vi "4461 - Create IO Channels Parallel Uneven array.vi"(0 "sample mode":i32(ring)=10178 items=["Finite Samples"=10178, "Continuous Samples"=10123], 1 "Channels: Lockin":T1={"REF f (Hz)"=[0.4, 0.4], "REF phi (deg)"=[0.0, 0.0]} {"REF phi (deg)" format="%#_3g"}, 6 "error in":errorcluster, 7 "AI Buffer Size (S)":i32=10, 8 "sampling info":cluster{"Fs":dbl, "#s":dbl}, 9 "AO":T2={"AO amp (V)"=[0.1, 0.09, 0.08, 0.07, 0.06, 0.05, 0.04, 0.03], "AO DC (V)"=[0.0, 0.0, 0.0, 0.0, 0.0, 0.0, 0.0, 0.0], "AO f (Hz)"=[13.0, 13.0, 13.0, 13.0, 13.0, 13.0, 13.0, 13.0], "AO phi (deg)"=[0.0, 0.0, 0.0, 0.0, 0.0, 0.0, 0.0, 0.0], "function"=[enum."Sine Wave", enum."Sine Wave", enum."Sine Wave", enum."Sine Wave", enum."Sine Wave", enum."Sine Wave", enum."Sine Wave", enum."Sine Wave"]} {"AO DC (V)" format="%#_6p"; "AO amp (V)" format="%#_6p"}, 10 "AO Configuration":T3(array[cluster]), 11 "AI Configuration":T4(array[cluster])) -> (2 "AO Task":refnum<k21>[](array[refnum]), 3 "AI task":refnum<k21>[](array[refnum]), 4 "error out":errorcluster, 5 "phase log":dbl[](array[numeric])=[0.99999999999938, 0.99999999999938])   [LabVIEW 2016]
uses:
  <vilib>/DAQmx/write.llb/DAQmx Write (Analog 1D Wfm NChan NSamp).vi
  <vilib>/DAQmx/read.llb/DAQmx Read (Analog 1D Wfm NChan NSamp).vi
  <vilib>/DAQmx/create/channels.llb/DAQmx Create Channel (AI-Voltage-Basic).vi
  <vilib>/DAQmx/configure/timing.llb/DAQmx Timing (Sample Clock).vi
  <vilib>/DAQmx/create/channels.llb/DAQmx Create Channel (AO-Voltage-Basic).vi
  <vilib>/DAQmx/miscellaneous.llb/DAQmx Fill In Error Info.vi
  <resource>/objmgr/daqmx.rc
panel:
  out "RefClk.Src":tag
  out "#samp":dbl
  in  "AI.FilterDelay":dbl
  in  "AI.Gain":dbl
  in  "input terminal configuration":i32(ring)=-1 items=["default"=-1, "RSE"=10083, "NRSE"=10078, "Differential"=10106, "Pseudodifferential"=12529]
  in  "output terminal configuration":i32(ring)=-1 items=["Default"=-1, "RSE"=10083, "Differential"=10106, "Pseudodifferential"=12529]
  out "SampClk.Timebase.Rate":dbl
  out "SampQuant.SampPerChan":dbl
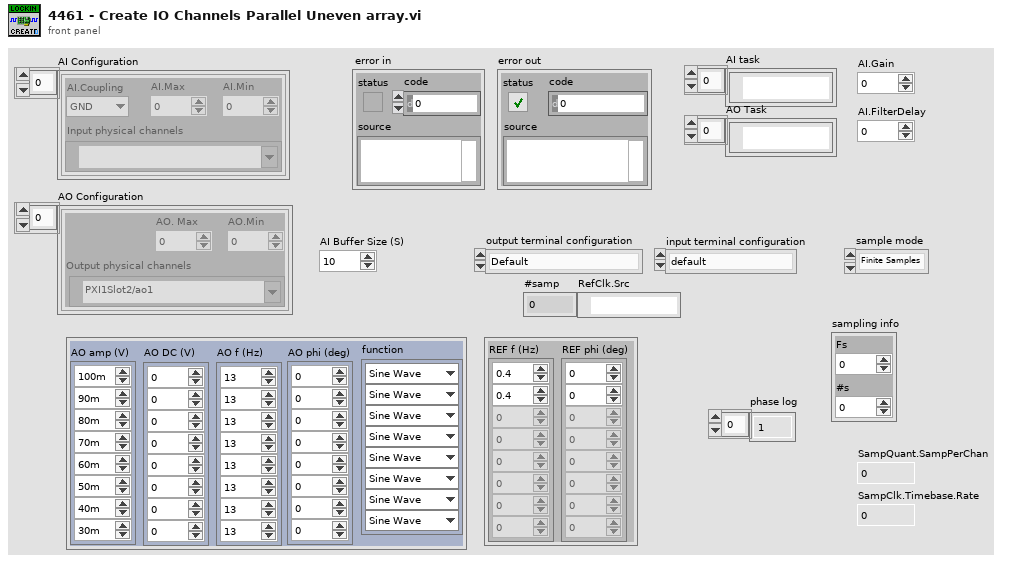
[diagram p1: front panel]
types:
  T1 = cluster{"REF f (Hz)":dbl[], "REF phi (deg)":dbl[]}
  T2 = cluster{"AO amp (V)":dbl[], "AO DC (V)":dbl[], "AO f (Hz)":dbl[], "AO phi (deg)":dbl[], "function":enum16{"Sine Wave", "Triangle Wave", "Square Wave", "Sawtooth Wave"}[]}
  T3 = cluster{"Output physical channels":tag, "AO. Max":dbl, "AO.Min":dbl}[]
  T4 = cluster{"AI.Coupling":enum16{"AC", "DC", "GND"}, "AI.Max":dbl, "AI.Min":dbl, "Input physical channels":tag}[]
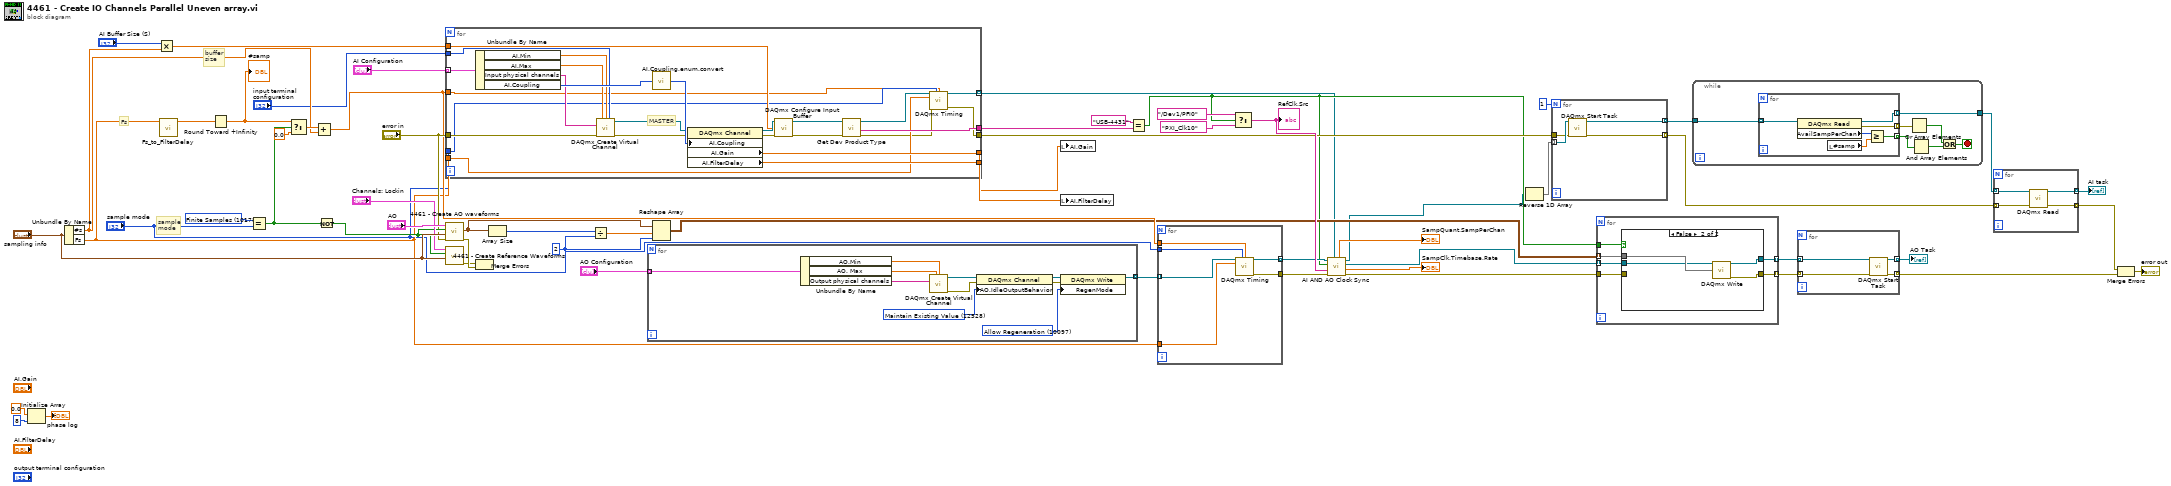
[diagram p0: block diagram]
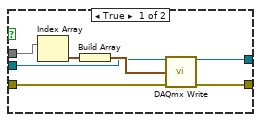
[diagram p2: hidden frame]
diagram:
  w14 = 2 ("y")
  w53 = 10178 items=["Finite Samples"=10178, "Continuous Samples"=10123] ("sample mode 2")
  # "Fs"
  # "sample\nmode"
  # "buffer\nsize"
  n1 = Initialize Array(0.0 ("element"), 8 ("dimension size")) -> (→"phase log":dbl[])
  n2 = Unbundle By Name("sampling info") -> ("#s"=w50:dbl, "Fs"=w29:dbl)
  n3 = Multiply(x="AI Buffer Size (S)", y=w50) -> (x*y=w36:dbl)
  n4 = call "Fs_to_FilterDelay.vi"("Fs"=w29) -> ("Total Filter Delay (samples)"=w56:dbl)  [unwired: 10 in]
  n5 = Round Toward +Infinity(x=w56) -> (ceil(x): smallest int >= x=w46:dbl)
  "#samp" <- w46
  n6 = Equal?(x=w53, y="sample mode") -> (x = y?=w48:bool)
  n7 = Select(t=w46, s=w48, f=0.0) -> (s? t:f=w54:dbl)
  n8 = Add(x=w54, y=w50) -> (x+y=w30:dbl)
  n9 = Not(x=w48) -> (.not. x?=w47:bool)
  n10 = for {
    tunnel: "AI Configuration" -> [w78] mode=indexing
    tunnel: "input terminal configuration" -> [w77]
    tunnel: [w76] -> w39
    tunnel: [w75] -> w38
    tunnel: "error in" -> [w74]
    tunnel: [w61] -> w7
    tunnel: w36 -> [w72]
    tunnel: [w68] -> w35
    tunnel: w29 -> [w66]
    tunnel: "sample mode" -> [w65]
    tunnel: w30 -> [w64]
    tunnel: [w63] -> w5 mode=indexing
    # "MASTER"
    n11 = Unbundle By Name(w78) -> ("AI.Min"=w83:dbl, "AI.Max"=w82:dbl, "Input physical channels"=w79:tag, "AI.Coupling"=w84:enum16{"AC", "DC", "GND"})
    n12 = call-poly <vilib>:"DAQmx Create Virtual Channel.vi"("maximum value"=w82, "minimum value"=w83, "input terminal configuration"=w77, "physical channels"=w79, "error in"=w74) -> ("task out"=w80:refnum<k21>, "error out"=w81:errorcluster)  [unwired: 9 in]
    n13 = call "AI.Coupling.enum.convert.vi"("AI.Coupling"=w84) -> ("Numeric"=w85:i32)
    n14 = property class="DAQmx Channel"(reference=w80, error in=w81, "AI.Coupling"=w85) -> (reference out=w73:refnum<k21>, error out=w69:errorcluster, "AI.Gain"=w75:dbl, "AI.FilterDelay"=w76:dbl)
    n15 = call <vilib>:"DAQmx Configure Input Buffer.vi"("task/channels in"=w73, "buffer size (in samples per channel)"=w72, "error in"=w69) -> ("task out"=w71:refnum<k21>, "error out"=w70:errorcluster)  [unwired: 11 in]
    n16 = call "Get Dev Product Type.vi"("error in (no error)"=w70, "Refnum in"=w71) -> ("error out"=w62:errorcluster, "ProductType"=w68:string, "Refnum out"=w67:refnum<k21>)  [unwired: 7 in]
    n17 = call-poly <vilib>:"DAQmx Timing.vi"("task/channels in"=w67, "sample mode"=w65, "samples per channel"=w64, "rate"=w66, "error in"=w62) -> ("task out"=w63:refnum<k21>, "error out"=w61:errorcluster)  [unwired: 9 in]
  }
  n18 = call "4461 - Create AO waveforms.vi"("error in (no error)"="error in", "sampling info"="sampling info", "reset signal"=w47, "AO"="AO") -> ("error out"=w42:errorcluster, "AO Array"=w27:waveform(dbl)[])  [unwired: 4 in, 2 out]
  n19 = call "4461 - Create Reference Waveforms.vi"("sampling info"="sampling info", "reset signal"=w47, "Lockin"="Channels: Lockin") -> ("error out"=w20:errorcluster)  [unwired: 5 in, 3 out]
  n20 = Merge Errors(w20, w42) -> ()  [unwired: 1 out]
  n21 = Array Size(array=w27) -> (size(s)=w26:i32)
  n22 = Divide(x=w26, y=w14) -> (x/y=w25:dbl)
  n23 = for {
    tunnel: "AO Configuration" -> [w87] mode=indexing
    tunnel: [w86] -> w31 mode=indexing
    w89 = 10097 items=["Allow Regeneration"=10097, "Do Not Allow Regeneration"=10158] ("RegenMode")
    w88 = 12528 items=["Zero Volts"=12526, "High-Impedance"=12527, "Maintain Existing Value"=12528] ("AO.IdleOutputBehavior")
    n24 = Unbundle By Name(w87) -> ("AO.Min"=w94:dbl, "AO. Max"=w95:dbl, "Output physical channels"=w96:tag)
    n25 = call-poly <vilib>:"DAQmx Create Virtual Channel.vi"("maximum value"=w95, "minimum value"=w94, "physical channels"=w96) -> ("task out"=w93:refnum<k21>, "error out"=w92:errorcluster)  [unwired: 11 in]
    n26 = property class="DAQmx Channel"(reference=w93, error in=w92, "AO.IdleOutputBehavior"=w88) -> (reference out=w91:refnum<k21>, error out=w90:errorcluster)
    n27 = property class="DAQmx Write"(reference=w91, error in=w90, "RegenMode"=w89) -> (reference out=w86:refnum<k21>)  [unwired: 1 out]
  }
  n28 = Reshape Array(w27, w25, w14) -> (w24:waveform(dbl)[][])
  n29 = local write "AI.Gain"(w38) -> ()
  n30 = local write "AI.FilterDelay"(w39) -> ()
  n31 = Equal?(x="USB-4431" ("ProductType"), y=w35) -> (x = y?=w6:bool)
  n32 = for {
    tunnel: w31 -> [w102] mode=indexing
    tunnel: [w101] -> w18 mode=indexing
    tunnel: w30 -> [w100]
    tunnel: w29 -> [w99]
    tunnel: "sample mode" -> [w98]
    tunnel: [w97] -> w15
    n33 = call-poly <vilib>:"DAQmx Timing.vi"("task/channels in"=w102, "sample mode"=w98, "samples per channel"=w100, "rate"=w99) -> ("task out"=w101:refnum<k21>, "error out"=w97:errorcluster)  [unwired: 10 in]
  }
  n34 = Select(t=tag "/Dev1/PFI0" ("RefClk.Src"), s=w6, f=tag "PXI_Clk10" ("RefClk.Src")) -> (s? t:f=w34:tag)
  "RefClk.Src" <- w34
  n35 = call "AI AND AO Clock Sync.vi"("AI In"=w5, "error in (no error)"=w15, "RefClk.Src"=w34, "USB-4431?"=w6, "AO in"=w18) -> ("error out"=w16:errorcluster, "SampClk.Timebase.Rate"=→"SampClk.Timebase.Rate":dbl, "AO Out"=w17:refnum<k21>[], "AI Out"=w4:refnum<k21>[], "SampQuant.SampPerChan"=→"SampQuant.SampPerChan":dbl)  [unwired: 2 in]
  n36 = Reverse 1D Array(array=w4) -> (reversed array=w3:refnum<k21>[])
  n37 = for {
    N: 1 -> [_]
    tunnel: w3 -> [w106] mode=indexing
    tunnel: [w103] -> w8 mode=indexing
    tunnel: w7 -> [w105]
    tunnel: [w104] -> w2 mode=indexing
    n38 = call <vilib>:"DAQmx Start Task.vi"("task/channels in"=w106, "error in"=w105) -> ("task out"=w104:refnum<k21>, "error out"=w103:errorcluster)  [unwired: 12 in]
  }
  n39 = for {
    tunnel: w24 -> [w112] mode=indexing
    tunnel: [w111] -> w23 mode=indexing
    tunnel: [w110] -> w22 mode=indexing
    tunnel: w17 -> [w109] mode=indexing
    tunnel: w16 -> [w108]
    tunnel: w6 -> [w107]
    n40 = case shown="False" w107 {
      tunnel: w112 -> [w119 w123]
      tunnel: [w117 w122] -> w111
      tunnel: [w116 w121] -> w110
      tunnel: w109 -> [w114 w120]
      tunnel: w108 -> [w113 _]
      frame True {
        n41 = Index Array(array=w119) -> (element=w118:waveform(dbl))  [unwired: 1 in]
        n42 = Build Array(w118) -> (w115:waveform(dbl)[])
        n43 = call-poly <vilib>:"DAQmx Write.vi"("task/channels in"=w114, "data"=w115, "error in"=w113) -> ("task out"=w117:refnum<k21>, "error out"=w116:errorcluster)  [unwired: 10 in, 1 out]
      }
      frame False {
        n44 = call-poly <vilib>:"DAQmx Write.vi"("task/channels in"=w120, "data"=w123) -> ("task out"=w122:refnum<k21>, "error out"=w121:errorcluster)  [unwired: 11 in, 1 out]
      }
    }
  }
  n45 = while {
    tunnel: w2 -> [w130]
    tunnel: [w124] -> w33
    stop <- w125 stop-if-true
    n46 = for {
      tunnel: w130 -> [w136] mode=indexing
      tunnel: [w133] -> w129 mode=indexing
      tunnel: [w132] -> w128 mode=indexing
      tunnel: [w131] -> w124 mode=indexing
      n47 = property class="DAQmx Read"(reference=w136) -> (reference out=w131:refnum<k21>, error out=w133:errorcluster, "AvailSampPerChan"=w135:u32)  [unwired: 1 in]
      n48 = local read "#samp"() -> (w134:dbl)
      n49 = Greater Or Equal?(x=w135, y=w134) -> (x >= y?=w132:bool)
    }
    n50 = Or Array Elements(Boolean array=w129) -> (logical OR=w126:bool)
    n51 = And Array Elements(Boolean array=w128) -> (logical AND=w127:bool)
    n52 = Or(x=w126, y=w127) -> (x .or. y?=w125:bool)
  }
  n53 = for {
    tunnel: w23 -> [w140] mode=indexing
    tunnel: w22 -> [w139] mode=indexing
    tunnel: [w138] -> w21 mode=indexing
    tunnel: [w137] -> w10 mode=indexing
    n54 = call <vilib>:"DAQmx Start Task.vi"("task/channels in"=w140, "error in"=w139) -> ("task out"=w138:refnum<k21>, "error out"=w137:errorcluster)  [unwired: 12 in]
  }
  "AO Task" <- w21
  n55 = for {
    tunnel: w33 -> [w144] mode=indexing
    tunnel: [w143] -> w32 mode=indexing
    tunnel: [w142] -> w9 mode=indexing
    tunnel: w8 -> [w141] mode=indexing
    n56 = call-poly <vilib>:"DAQmx Read.vi"("task/channels in"=w144, "error in"=w141) -> ("task out"=w143:refnum<k21>, "error out"=w142:errorcluster)  [unwired: 11 in, 1 out]
  }
  "AI task" <- w32
  n57 = Merge Errors(w9, w10) -> (→"error out":errorcluster)
